vi "Get Server Certificates (Client).vi"(10 "Server Certificates":T1) -> (2 "trusted server certificates":path[](array[path]))   [LabVIEW 2013, in "OPC UA Server runtime.lvclass"]
doc: "Get paths to trusted server certificates used in creating an OPC UA Client connection"
uses:
  OPC UA Server runtime.lvclass
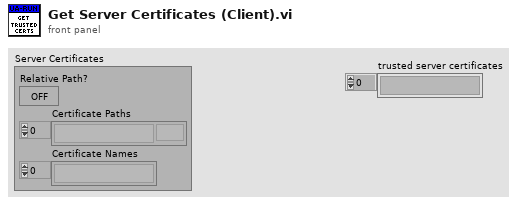
[diagram p1: front panel]
types:
  T1 = cluster{"Relative Path?":bool, "Certificate Paths":path[], "Certificate Names":string[]}
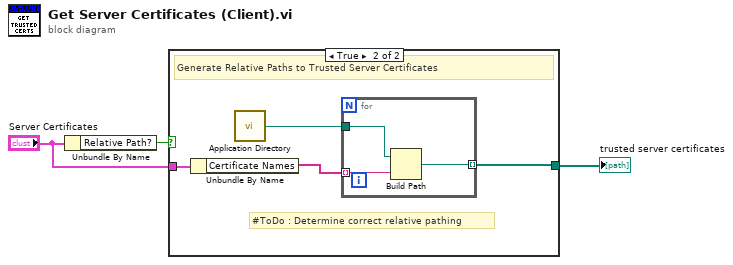
[diagram p0: block diagram]
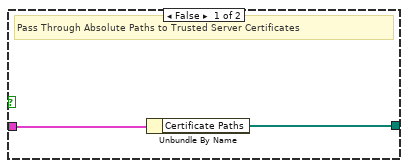
[diagram p2: hidden frame]
diagram:
  n1 = Unbundle By Name("Server Certificates") -> ("Relative Path?"=w3:bool)
  n2 = case shown="True" w3 {
    tunnel: "Server Certificates" -> [w5 w9]
    tunnel: [w4 w7] -> w1
    frame False {
      # "Pass Through Absolute Paths to Trusted Server Certificates"
      n3 = Unbundle By Name(w5) -> ("Certificate Paths"=w4:path[])
    }
    frame True {
      # "#ToDo : Determine correct relative pathing"
      # "Generate Relative Paths to Trusted Server Certificates"
      n4 = Unbundle By Name(w9) -> ("Certificate Names"=w8:string[])
      n5 = call <vilib>:"Application Directory.vi"() -> ("Application Directory"=w6:path)
      n6 = for {
        tunnel: w8 -> [w12] mode=indexing
        tunnel: [w11] -> w7 mode=indexing
        tunnel: w6 -> [w10]
        n7 = Build Path(base path=w10, name or relative path=w12) -> (appended path=w11:path)
      }
    }
  }
  "trusted server certificates" <- w1
